vi "zaxpy - Scalar-Vector Product (CDB).vi"(5 "yInc":i32=1, 6 "alpha":cdb=1.0+0.0i, 7 "xInc":i32=1, 10 "y":cdb[](array[numeric]), 11 "x":cdb[](array[numeric])) -> (0 "error":i32, 3 "zaxpy":cdb[](array[numeric]))   [LabVIEW 2020, in "NI_AALBLAS.lvlib"]
doc: "Calculates the product of a scalar and a vector."
uses:
  <vilib>/Analysis/NI_AALBLAS.lvlib
  <vilib>/Analysis/BLAS.llb/Fucntion.ctl
  <vilib>/Analysis/BLAS.llb/BLAS1 Utility(CDB).vi
panel:
  # "zaxpy=alpha*x+y"
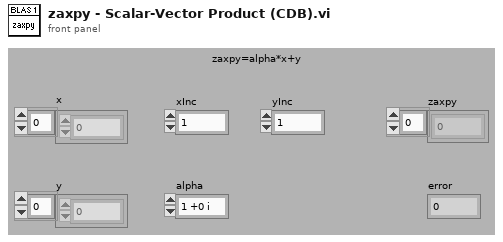
[diagram p1: front panel]
types:
  T1 = typedef "NI_AALBLAS.lvlib/Fucntion.ctl" = u16
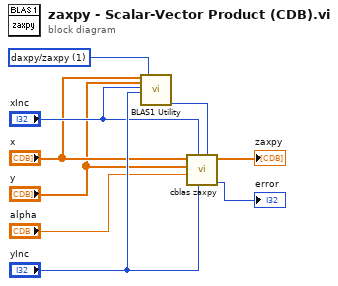
[diagram p0: block diagram]
diagram:
  w2 = T1 1 items=["ddot/zdotu/zdotc", "daxpy/zaxpy", "dnrm2/dznrm2", "dasum/dzasum", "dcopy/zcopy", "dswap/zswap", "drotm", "drot/zdrot", "idamax/izamax", "idamin/izamin", "dgemv/zgemv", "dsymv/zhemv", "dtrmv/ztrmv", "dsyr/zher", "dsyr2/zher2", "dger/zgeru/zgerc", "dtrsv/ztrsv", "dgemm/zgemm", "dsymm/zsymm/zhemm", "dtrmm/ztrmm", "dsyrk/zsyrk/zherk", "dsyr2k/zsyr2k/zher2k", "dtrsm/ztrsm"] ("function")
  n1 = call-poly <vilib>:"BLAS1 Utility.vi"("x"="x", "y"="y", "xInc"="xInc", "yInc"="yInc", "function"=w2) -> ("n"=w1:i32)  [unwired: 14 out]
  n2 = call <vilib>:"cblas zaxpy.vi"("n"=w1, "incy"="yInc", "incx"="xInc", "alpha"="alpha", "y"="y", "x"="x") -> ("error"=→"error":i32, "zaxpy"=→"zaxpy":cdb[])  [unwired: 4 out]
